vi "Begin.vi"(8 "error in":errorcluster) -> (0 "error out":errorcluster)   [LabVIEW 2016]
doc: "Called before other user functions, this VI is expected to open initial I/O refnums, load in file data, and do all program initialization. Notice that the <B>error out</B> terminal is simply used for data flow. Wiring it to other structures or subVIs ensures that this VI runs first."
uses:
  <vilib>/Rock Robotics/WPI/DriverStation/WPI_DriverStationRobotMode2.ctl
  <vilib>/Rock Robotics/WPI/Joystick/WPI_JoystickDeviceEnum.ctl
  <vilib>/Rock Robotics/SystemInterfaces/DIO/FPGA_DIOChannel.ctl
  <vilib>/Rock Robotics/WPI/ThirdParty/CanMotor/TalonSRX/WPI_CANTalonSRX_FeedbackSelect.ctl
  <vilib>/Rock Robotics/WPI/ThirdParty/CanMotor/TalonSRX/WPI_CANTalonSRX_APIControlMode.ctl
  <vilib>/Rock Robotics/SystemInterfaces/DIO/FPGA_DIOPWMChannel.ctl
  Robot Global Data.vi
  <vilib>/Rock Robotics/WPI/MotorControl/WPI_MotorControlOpen SPARK.vi
  <vilib>/Rock Robotics/WPI/Switch/WPI_SwitchOpenLimit.vi
  <vilib>/Rock Robotics/WPI/Solenoid/WPI_SolenoidOpenSingle.vi
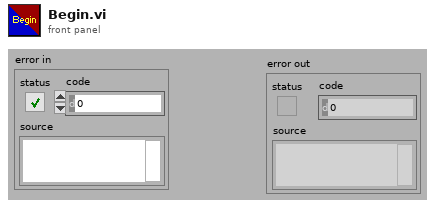
[diagram p1: front panel]
types:
  T1 = enum16{"PWM 0", "PWM 1", "PWM 2", "PWM 3", "PWM 4", "PWM 5", "PWM 6", "PWM 7", "PWM 8", "PWM 9"}
  T2 = typedef "FPGA_DIOPWMChannel.ctl" = enum8{"PWM 0", "PWM 1", "PWM 2", "PWM 3", "PWM 4", "PWM 5", "PWM 6", "PWM 7", "PWM 8", "PWM 9", "PWM MXP 0", "PWM MXP 1", "PWM MXP 2", "PWM MXP 3", "PWM MXP 4", "PWM MXP 5", "PWM MXP 6", "PWM MXP 7", "PWM MXP 8", "PWM MXP 9", "Invalid"}
  T3 = typedef "FPGA_DIOChannel.ctl" = enum8{"DIO 0", "DIO 1", "DIO 2", "DIO 3", "DIO 4", "DIO 5", "DIO 6", "DIO 7", "DIO 8", "DIO 9", "DIO MXP 0", "DIO MXP 1", "DIO MXP 2", "DIO MXP 3", "DIO MXP 4", "DIO MXP 5", "DIO MXP 6", "DIO MXP 7", "DIO MXP 8", "DIO MXP 9", "DIO MXP 10", "DIO MXP 11", "DIO MXP 12", "DIO MXP 13", "DIO MXP 14", "DIO MXP 15", "SPI Port CS1", "SPI Port CS2", "SPI Port CS3", "SPI Port MISO", "SPI Port MOSI", "Invalid"}
  T4 = enum16{"Solenoid 0", "Solenoid 1", "Solenoid 2", "Solenoid 3", "Solenoid 4", "Solenoid 5"}
  T5 = typedef "WPI_CANTalonSRX_FeedbackSelect.ctl" = u8
  T6 = typedef "WPI_CANTalonSRX_APIControlMode.ctl" = enum8{"Percent VBus", "Speed", "Position", "Slave", "Unchanged / Invalid", "Voltage Compensation", "Current", "Motion Profile", "Motion Magic"}
  T7 = typedef "WPI_JoystickDeviceEnum.ctl" = enum16{"USB 0", "USB 1", "USB 2", "USB 3", "USB 4", "USB 5"}
  T8 = typedef "WPI_DriverStationRobotMode2.ctl" = enum16{"Autonomous Disabled", "Autonomous Enabled", "Teleop Disabled", "Teleop Enabled", "Disconnected", "Finish", "Test Disabled", "Test Enabled", "Emergency Stopped"}
  T9 = typedef "WPI_MotorControlDeviceRef.ctl" = cluster{"DeviceStatus":errorcluster, "Type":T10, "PWM":cluster{"PWM Channel":T2, "DeadBand":T11}, "CAN":cluster{"Device Number":u8, "SetOutput VI Ref":variant, "GetOutput VI Ref":variant, "Enable VI Ref":variant, "Disable VI Ref":variant, "Data":variant}, "Invert":bool}
  T10 = typedef "WPI_MotorControlType.ctl" = enum16{"PWM", "CAN"}
  T11 = typedef "WPI_PWMDeadband.ctl" = cluster{"Name":string, "maxPositivePwm":i32, "minPositivePwm":i32, "centerPwm":i32, "maxNegativePwm":i32, "minNegativePwm":i32, "angularRange":u16}
  T12 = typedef "WPI_CANTalonSRX_GlobalStatus.ctl" = cluster{"Applied Throttle":dbl, "Module Enabled":bool, "CAN Error":errorcluster, "Closed Loop Error":dbl, "Forward Limit Switch Closed":bool, "Reverse Limit Switch Closed":bool, "Sensor Position":dbl, "Sensor Velocity":dbl, "Current":dbl, "Sticky Fault - Over Temp":bool, "Sticky Fault - Under Voltage":bool, "Sticky Fault - Forward Limit":bool, "Sticky Fault - Reverse Limit":bool, "Sticky Fault - Forward Soft Limit":bool, "Sticky Fault - Reverse Soft Limit":bool, "Brake is Enabled":bool, "Encoder Position":dbl, "Encoder Velocity":dbl, "Encoder Index Count":dbl, "Encoder A Pin State":bool, "Encoder B Pin State":bool, "Encoder Index Pin State":bool, "Analog In":dbl, "Analog In Velocity":dbl, "Temperature (C)":dbl, "Battery Voltage":dbl, "Control 5 Is Supported":bool, "Current Profile Slot Select":dbl, "Pos Div 8":bool, "Vel Div 4":bool, "Pulse Width Position":i32, "Pulse Width Velocity":i32, "Pulse Width Rise To Rise (us)":i32, "Pulse Width Rise To Fall (us)":i32, "Mot Prof Active Is Under Run":bool, "Mot Prof Active Has Under Run":bool, "Mot Prof Active Is Last":bool, "Mot Prof Active Velocity Only":bool, "Mot Prof Active Is Valid":bool, "Mot Prof Buffer Is Full":bool, "Mot Prof Active Profile Slot Select":i32, "Mot Prof NextID":i32, "Mot Prof Count":i32, "Mot Prof Active Velocity":dbl, "Mot Prof Active Position":dbl, "Mot Prof Output Enable":i32}
  T13 = typedef "WPI_SwitchDevRef.ctl" = cluster{"DevStatus":errorcluster, "DIO Channel":T3, "CntIndex":T14, "Normally Closed":bool}
  T14 = typedef "FPGA_CounterCtrSystemIndex.ctl" = enum8{"Ctr 0", "Ctr 1", "Ctr 2", "Ctr 3", "Ctr 4", "Ctr 5", "Ctr 6", "Ctr 7", "Invalid"}
  T15 = typedef "WPI_DigitalOutputDevRef.ctl" = cluster{"DIO Channel":T3, "DevStatus":errorcluster}
  T16 = typedef "WPI_ServoDeviceRef.ctl" = cluster{"DeviceStatus":errorcluster, "PWM Channel":T2, "DeadBand":T11}
  T17 = typedef "WPI_JoystickDevRef.ctl" = cluster{"Device":T7}
  T18 = typedef "WPI_SolenoidDevRef.ctl" = cluster{"DevStatus":errorcluster, "Pneumatics Control Module":u8, "Forward Solenoid Channel":T19, "Reverse Solenoid Channel":T19}
  T19 = typedef "WPI_SolenoidChannel.ctl" = enum8{"Solenoid 0", "Solenoid 1", "Solenoid 2", "Solenoid 3", "Solenoid 4", "Solenoid 5", "Solenoid 6", "Solenoid 7", "Invalid"}
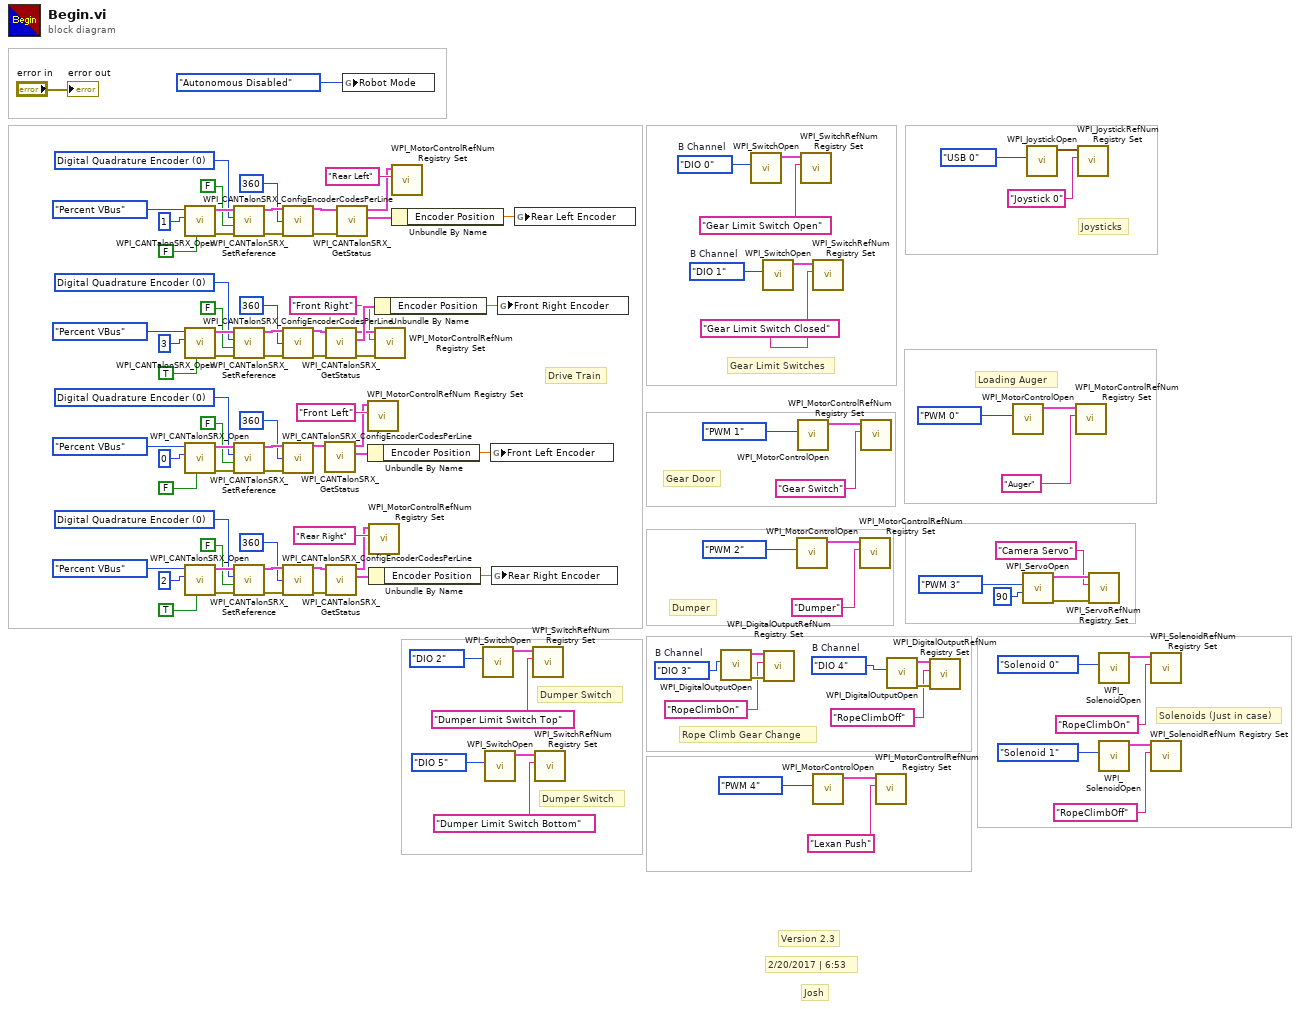
[diagram p0: block diagram]
diagram:
  w18 = FPGA_DIOChannel."DIO 4"  # B Channel
  w19 = FPGA_DIOChannel."DIO 3"  # B Channel
  w55 = T5 0 items=["Digital Quadrature Encoder"=0, "Analog Pot"=2, "Analog Encoder"=3, "Count on Quad-A (Rising-Edge)"=4, "Count on Quad-A (Falling-Edge)"=5, "Position is Pulse-Width"=8] ("Talon SRX Feedback Select")
  w65 = T5 0 items=["Digital Quadrature Encoder"=0, "Analog Pot"=2, "Analog Encoder"=3, "Count on Quad-A (Rising-Edge)"=4, "Count on Quad-A (Falling-Edge)"=5, "Position is Pulse-Width"=8] ("Talon SRX Feedback Select")
  w74 = T5 0 items=["Digital Quadrature Encoder"=0, "Analog Pot"=2, "Analog Encoder"=3, "Count on Quad-A (Rising-Edge)"=4, "Count on Quad-A (Falling-Edge)"=5, "Position is Pulse-Width"=8] ("Talon SRX Feedback Select")
  w84 = T5 0 items=["Digital Quadrature Encoder"=0, "Analog Pot"=2, "Analog Encoder"=3, "Count on Quad-A (Rising-Edge)"=4, "Count on Quad-A (Falling-Edge)"=5, "Position is Pulse-Width"=8] ("Talon SRX Feedback Select")
  w91 = FPGA_DIOChannel."DIO 0"  # B Channel
  w94 = FPGA_DIOChannel."DIO 1"  # B Channel
  # "Josh"
  # "Dumper Switch"
  # "Solenoids (Just in case)"
  # "Rope Climb Gear Change"
  # "Dumper Switch"
  # "Gear Limit Switches"
  # "Joysticks"
  # "Dumper"
  # "Loading Auger"
  # "Drive Train"
  # "Gear Door"
  # "Version 2.3"
  # "2/20/2017 | 6:53"
  n1 = call <vilib>:"WPI_CANTalonSRX_Open.vi"("Invert"=FALSE, "Device Number"=u8 1, "Control Mode"=WPI_CANTalonSRX_APIControlMode."Percent VBus") -> ("error out"=w77:errorcluster, "CAN Talon SRX Ref"=w80:T9)  [unwired: 7 in]
  n2 = call <vilib>:"WPI_CANTalonSRX_Open.vi"("Invert"=TRUE, "Device Number"=u8 3, "Control Mode"=WPI_CANTalonSRX_APIControlMode."Percent VBus") -> ("error out"=w68:errorcluster, "CAN Talon SRX Ref"=w71:T9)  [unwired: 7 in]
  n3 = call <vilib>:"WPI_CANTalonSRX_Open.vi"("Invert"=FALSE, "Device Number"=u8 0, "Control Mode"=WPI_CANTalonSRX_APIControlMode."Percent VBus") -> ("error out"=w58:errorcluster, "CAN Talon SRX Ref"=w61:T9)  [unwired: 7 in]
  n4 = call <vilib>:"WPI_CANTalonSRX_Open.vi"("Invert"=TRUE, "Device Number"=u8 2, "Control Mode"=WPI_CANTalonSRX_APIControlMode."Percent VBus") -> ("error out"=w87:errorcluster, "CAN Talon SRX Ref"=w90:T9)  [unwired: 7 in]
  n5 = call <vilib>:"WPI_CANTalonSRX_SetReference.vi"("error in (no error)"=w77, "Reverse Feedback Sensor"=FALSE, "Feedback Reference"=w74, "CAN Talon SRX Ref"=w80) -> ("error out"=w78:errorcluster, "CAN Talon SRX Ref"=w79:T9)  [unwired: 6 in]
  n6 = call <vilib>:"WPI_CANTalonSRX_SetReference.vi"("error in (no error)"=w68, "Reverse Feedback Sensor"=FALSE, "Feedback Reference"=w65, "CAN Talon SRX Ref"=w71) -> ("error out"=w69:errorcluster, "CAN Talon SRX Ref"=w70:T9)  [unwired: 6 in]
  n7 = call <vilib>:"WPI_CANTalonSRX_SetReference.vi"("error in (no error)"=w58, "Reverse Feedback Sensor"=FALSE, "Feedback Reference"=w55, "CAN Talon SRX Ref"=w61) -> ("error out"=w59:errorcluster, "CAN Talon SRX Ref"=w60:T9)  [unwired: 6 in]
  n8 = call <vilib>:"WPI_CANTalonSRX_SetReference.vi"("error in (no error)"=w87, "Reverse Feedback Sensor"=FALSE, "Feedback Reference"=w84, "CAN Talon SRX Ref"=w90) -> ("error out"=w88:errorcluster, "CAN Talon SRX Ref"=w89:T9)  [unwired: 6 in]
  n9 = call <vilib>:"WPI_CANTalonSRX_ConfigEncoderCodesPerLine.vi"("CAN Talon SRX Ref"=w79, "Number Encoder Lines\n(Counts Per Rotation)"=360, "error in (no error)"=w78) -> ("CAN Talon SRX Ref"=w53:T9, "error out"=w54:errorcluster)  [unwired: 11 in]
  n10 = call <vilib>:"WPI_CANTalonSRX_ConfigEncoderCodesPerLine.vi"("CAN Talon SRX Ref"=w70, "Number Encoder Lines\n(Counts Per Rotation)"=360, "error in (no error)"=w69) -> ("CAN Talon SRX Ref"=w46:T9, "error out"=w45:errorcluster)  [unwired: 11 in]
  n11 = call <vilib>:"WPI_CANTalonSRX_ConfigEncoderCodesPerLine.vi"("CAN Talon SRX Ref"=w60, "Number Encoder Lines\n(Counts Per Rotation)"=360, "error in (no error)"=w59) -> ("CAN Talon SRX Ref"=w49:T9)  [unwired: 11 in, 1 out]
  n12 = call <vilib>:"WPI_CANTalonSRX_ConfigEncoderCodesPerLine.vi"("CAN Talon SRX Ref"=w89, "Number Encoder Lines\n(Counts Per Rotation)"=360, "error in (no error)"=w88) -> ("CAN Talon SRX Ref"=w41:T9, "error out"=w40:errorcluster)  [unwired: 11 in]
  n13 = call <vilib>:"WPI_CANTalonSRX_GetStatus.vi"("CAN Talon SRX Ref"=w49) -> ("Talon SRX Status"=w50:T12, "CAN Talon SRX Ref"=w48:T9)  [unwired: 8 in, 1 out]
  n14 = call <vilib>:"WPI_CANTalonSRX_GetStatus.vi"("error in (no error)"=w45, "CAN Talon SRX Ref"=w46) -> ("error out"=w43:errorcluster, "Talon SRX Status"=w47:T12, "CAN Talon SRX Ref"=w44:T9)  [unwired: 7 in]
  n15 = call <vilib>:"WPI_CANTalonSRX_GetStatus.vi"("error in (no error)"=w40, "CAN Talon SRX Ref"=w41) -> ("Talon SRX Status"=w38:T12, "CAN Talon SRX Ref"=w37:T9)  [unwired: 7 in, 1 out]
  n16 = call <vilib>:"WPI_CANTalonSRX_GetStatus.vi"("error in (no error)"=w54, "CAN Talon SRX Ref"=w53) -> ("Talon SRX Status"=w51:T12, "CAN Talon SRX Ref"=w52:T9)  [unwired: 7 in, 1 out]
  n17 = global write "Robot Global Data.vi" "Robot Mode"(WPI_DriverStationRobotMode2."Autonomous Disabled" ("Robot Mode")) -> ()
  n18 = call <vilib>:"WPI_MotorControlRefNum Registry Set.vi"("refnum name"="Front Left", "MotorControlDevRef"=w48) -> ()  [unwired: 8 in, 2 out]
  n19 = Unbundle By Name(w50) -> ("Encoder Position"=w36:dbl)
  n20 = call <vilib>:"WPI_MotorControlRefNum Registry Set.vi"("refnum name"="Rear Right", "MotorControlDevRef"=w37) -> ()  [unwired: 8 in, 2 out]
  n21 = Unbundle By Name(w38) -> ("Encoder Position"=w34:dbl)
  n22 = Unbundle By Name(w47) -> ("Encoder Position"=w33:dbl)
  n23 = call <vilib>:"WPI_MotorControlRefNum Registry Set.vi"("error in (no error)"=w43, "refnum name"="Front Right", "MotorControlDevRef"=w44) -> ()  [unwired: 7 in, 2 out]
  n24 = call <vilib>:"WPI_MotorControlRefNum Registry Set.vi"("refnum name"="Rear Left", "MotorControlDevRef"=w52) -> ()  [unwired: 8 in, 2 out]
  n25 = Unbundle By Name(w51) -> ("Encoder Position"=w35:dbl)
  n26 = call-poly <vilib>:"WPI_SwitchOpen.vi"("DIO Channel"=FPGA_DIOChannel."DIO 2") -> ("SwitchDevRef"=w28:T13)  [unwired: 9 in, 1 out]
  n27 = call-poly <vilib>:"WPI_SwitchOpen.vi"("DIO Channel"=FPGA_DIOChannel."DIO 5") -> ("SwitchDevRef"=w9:T13)  [unwired: 9 in, 1 out]
  n28 = global write "Robot Global Data.vi" "Front Left Encoder"(w36) -> ()
  n29 = global write "Robot Global Data.vi" "Rear Right Encoder"(w34) -> ()
  n30 = global write "Robot Global Data.vi" "Front Right Encoder"(w33) -> ()
  n31 = global write "Robot Global Data.vi" "Rear Left Encoder"(w35) -> ()
  n32 = call <vilib>:"WPI_SwitchRefNum Registry Set.vi"("refnum name"="Dumper Limit Switch Top", "SwitchDevRef"=w28) -> ()  [unwired: 8 in, 2 out]
  n33 = call <vilib>:"WPI_SwitchRefNum Registry Set.vi"("refnum name"="Dumper Limit Switch Bottom", "SwitchDevRef"=w9) -> ()  [unwired: 8 in, 2 out]
  n34 = call <vilib>:"WPI_DigitalOutputOpen.vi"("DIO Channel"=w19) -> ("error out"=w25:errorcluster, "DigitalOutputDevRef"=w24:T15)  [unwired: 9 in]
  n35 = call-poly <vilib>:"WPI_SwitchOpen.vi"("DIO Channel"=w91) -> ("SwitchDevRef"=w93:T13)  [unwired: 9 in, 1 out]
  n36 = call-poly <vilib>:"WPI_SwitchOpen.vi"("DIO Channel"=w94) -> ("SwitchDevRef"=w96:T13)  [unwired: 9 in, 1 out]
  n37 = call <vilib>:"WPI_DigitalOutputRefNum Registry Set.vi"("error in (no error)"=w25, "refnum name"="RopeClimbOn", "DigitalOutputDevRef"=w24) -> ()  [unwired: 7 in, 2 out]
  n38 = call-poly <vilib>:"WPI_MotorControlOpen.vi"("PWM Channel"=T1."PWM 2") -> ("MotorControlDeviceRef"=w101:T9)  [unwired: 9 in, 1 out]
  n39 = call-poly <vilib>:"WPI_MotorControlOpen.vi"("PWM Channel"=T1."PWM 1") -> ("MotorControlDeviceRef"=w99:T9)  [unwired: 9 in, 1 out]
  n40 = call <vilib>:"WPI_SwitchRefNum Registry Set.vi"("refnum name"="Gear Limit Switch Open", "SwitchDevRef"=w93) -> ()  [unwired: 8 in, 2 out]
  n41 = call <vilib>:"WPI_SwitchRefNum Registry Set.vi"("refnum name"="Gear Limit Switch Closed", "SwitchDevRef"=w96) -> ()  [unwired: 8 in, 2 out]
  n42 = call-poly <vilib>:"WPI_MotorControlOpen.vi"("PWM Channel"=T1."PWM 4") -> ("MotorControlDeviceRef"=w2:T9)  [unwired: 9 in, 1 out]
  n43 = call <vilib>:"WPI_MotorControlRefNum Registry Set.vi"("refnum name"="Dumper", "MotorControlDevRef"=w101) -> ()  [unwired: 8 in, 2 out]
  n44 = call <vilib>:"WPI_MotorControlRefNum Registry Set.vi"("refnum name"="Gear Switch", "MotorControlDevRef"=w99) -> ()  [unwired: 8 in, 2 out]
  n45 = call <vilib>:"WPI_MotorControlRefNum Registry Set.vi"("refnum name"="Lexan Push", "MotorControlDevRef"=w2) -> ()  [unwired: 8 in, 2 out]
  n46 = call <vilib>:"WPI_DigitalOutputOpen.vi"("DIO Channel"=w18) -> ("error out"=w22:errorcluster, "DigitalOutputDevRef"=w21:T15)  [unwired: 9 in]
  n47 = call <vilib>:"WPI_DigitalOutputRefNum Registry Set.vi"("error in (no error)"=w22, "refnum name"="RopeClimbOff", "DigitalOutputDevRef"=w21) -> ()  [unwired: 7 in, 2 out]
  n48 = call-poly <vilib>:"WPI_MotorControlOpen.vi"("PWM Channel"=T1."PWM 0") -> ("MotorControlDeviceRef"=w104:T9)  [unwired: 9 in, 1 out]
  n49 = call <vilib>:"WPI_ServoOpen.vi"("Angular Range"=u16 90, "PWM Channel"=FPGA_DIOPWMChannel."PWM 3") -> ("error out"=w7:errorcluster, "ServoDeviceRef"=w8:T16)  [unwired: 8 in]
  n50 = call <vilib>:"WPI_JoystickOpen.vi"("JoystickDevice"=WPI_JoystickDeviceEnum."USB 0") -> ("JoystickDevRef"=w110:T17)  [unwired: 10 in]
  n51 = call <vilib>:"WPI_MotorControlRefNum Registry Set.vi"("refnum name"="Auger", "MotorControlDevRef"=w104) -> ()  [unwired: 8 in, 2 out]
  n52 = call <vilib>:"WPI_JoystickRefNum Registry Set.vi"("refnum name"="Joystick 0", "JoystickDevRef"=w110) -> ()  [unwired: 8 in, 2 out]
  n53 = call <vilib>:"WPI_ServoRefNum Registry Set.vi"("error in (no error)"=w7, "refnum name"="Camera Servo", "ServoDeviceRef"=w8) -> ()  [unwired: 7 in, 2 out]
  n54 = call-poly <vilib>:"WPI_SolenoidOpen.vi"("Solenoid Channel"=T4."Solenoid 0") -> ("SolenoidDevRef"=w15:T18)  [unwired: 9 in, 1 out]
  n55 = call-poly <vilib>:"WPI_SolenoidOpen.vi"("Solenoid Channel"=T4."Solenoid 1") -> ("SolenoidDevRef"=w12:T18)  [unwired: 9 in, 1 out]
  n56 = call <vilib>:"WPI_SolenoidRefNum Registry Set.vi"("refnum name"="RopeClimbOn", "SolenoidDevRef"=w15) -> ()  [unwired: 8 in, 2 out]
  n57 = call <vilib>:"WPI_SolenoidRefNum Registry Set.vi"("refnum name"="RopeClimbOff", "SolenoidDevRef"=w12) -> ()  [unwired: 8 in, 2 out]
  "error out" <- "error in"
